vi "SRV_Return All After Last Match in String.vi"(7 "String":string, 9 "String to Match":string) -> (8 "Match Plus Remaining String":string)   [LabVIEW 2009]
doc: "Returns the last match of \"String to Match\" plus the remainder of the string following the last match.\n\n\nAuthor: Mike Schultz - Logic PD"
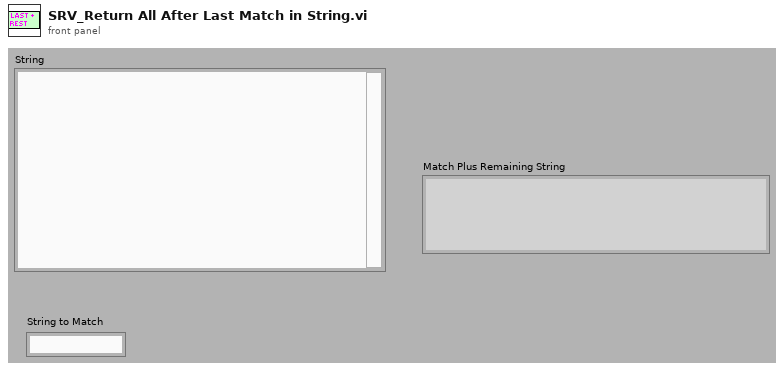
[diagram p1: front panel]
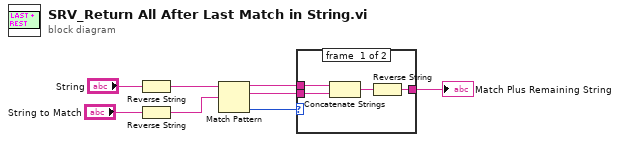
[diagram p0: block diagram]
diagram:
  n1 = Reverse String(1:"String") -> (0:w3:string)
  n2 = Reverse String(1:"String to Match") -> (0:w1:string)
  n3 = Match Pattern(string=w3, regular expression=w1) -> (before substring=w6:string, match substring=w7:string, offset past match=w4:i32)  [unwired: 1 in, 1 out]
  n4 = case shown="Default" w4 {
    tunnel: w7 -> [w12 _]
    tunnel: w6 -> [w11 _]
    tunnel: [w9 _] -> w5
    frame #0 {
      n5 = Concatenate Strings(w11, w12) -> (w10:string)
      n6 = Reverse String(1:w10) -> (0:w9:string)
    }
    frame #1 {
    }
  }
  "Match Plus Remaining String" <- w5
